vi "ProdaNG.Configurator.Popup.Delete.vi"(10 "Elements to delete":T1[](array[typedef])) -> (5 "OK?":bool)   [LabVIEW 2016]
uses:
  ProdaNG.Tree.Fglb.Data.ctl
  ProdaNG.Tree.Fglb.Element.ctl
panel:
  out "unblock time":timestamp
  in  "Button.Cancel":bool
  in  "Button.OK":bool
  out "Msg":string
  out "Elements":i32(listbox)
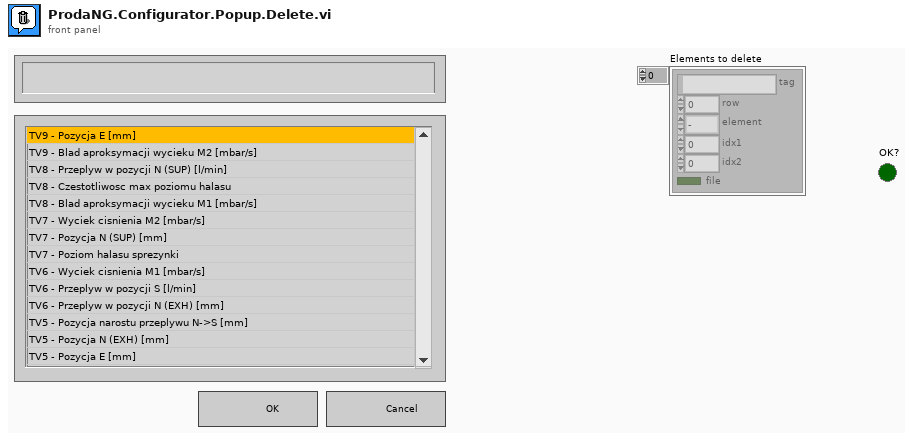
[diagram p1: front panel]
types:
  T1 = typedef "ProdaNG.Tree.Fglb.Data.ctl" = cluster{"tag":string, "row":i32, "element":T2, "idx1":i32, "idx2":i32, "file":bool}
  T2 = typedef "ProdaNG.Tree.Fglb.Element.ctl" = enum16{"-", "PP", "TS", "TP", "TV"}
  T3 = enum8{"Enabled", "Disabled", "Disabled and Grayed Out"}
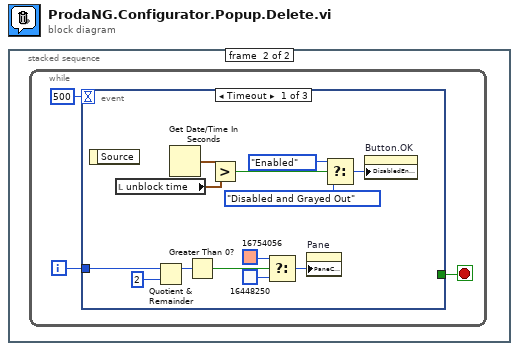
[diagram p0: block diagram]
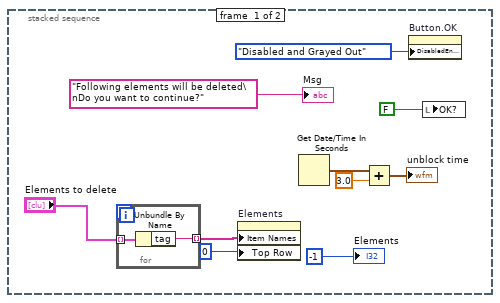
[diagram p2: hidden frame]
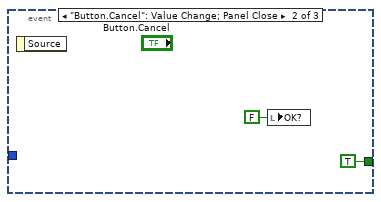
[diagram p3: hidden frame]
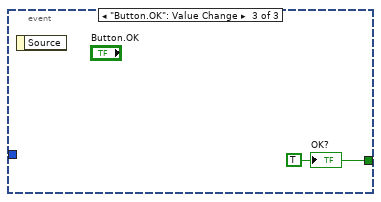
[diagram p4: hidden frame]
diagram:
  n1 = stacked-sequence {
    frame #0 {
      n2 = for {
        tunnel: "Elements to delete" -> [w12] mode=indexing
        tunnel: [w11] -> w7 mode=indexing
        n3 = Unbundle By Name(w12) -> ("tag"=w11:string)
      }
      n4 = property on="Elements" class="LstBox (strict)"("Item Names"=w7, "Top Row"=0) -> ()  [unwired: 2 in, 2 out]
      n5 = Get Date/Time In Seconds() -> (seconds since 1Jan1904=w3:timestamp)
      n6 = Add(x=w3, y=3.0) -> (x+y=→"unblock time":timestamp)
      n7 = property on="Button.OK" class="Bool"("DisabledEnum"=T3."Disabled and Grayed Out" ("Disabled")) -> ()  [unwired: 2 in, 2 out]
      n8 = local write "OK?"(FALSE ("OK?")) -> ()
      "Msg" <- "Following elements will be deleted\nDo you want to continue?" ("Msg")
      "Elements" <- -1 ("Elements")
    }
    frame #1 {
      n9 = while {
        i -> [w13]
        stop <- w15 stop-if-true
        n10 = event shown="[0] Timeout" {
          selector: _ -> [_ _ _]
          dyn-events: _ -> [_ _ _]
          timeout: 500 -> [_ _ _]
          tunnel: [_ TRUE ("OK?") w31] -> w15
          tunnel: w13 -> [w28 _ _]
          event Timeout {
            n11 = event-data() -> ()  [unwired: 1 in, 1 out]
            n12 = local read "unblock time"() -> (w21:timestamp)
            n13 = Quotient & Remainder(x=w28, y=2) -> (x-y*floor(x/y)=w26:i32)  [unwired: 1 out]
            n14 = Get Date/Time In Seconds() -> (seconds since 1Jan1904=w20:timestamp)
            n15 = Greater Than 0?(x=w26) -> (x > 0?=w25:bool)
            n16 = Greater?(x=w20, y=w21) -> (0:w19:bool)
            n17 = Select(t=u32 16754056, s=w25, f=u32 16448250) -> (s? t:f=w22:u32)
            n18 = property on="Pane" class="Pane"("PaneColor"=w22) -> ()  [unwired: 2 in, 2 out]
            n19 = Select(t=T3."Enabled" ("Disabled"), s=w19, f=T3."Disabled and Grayed Out" ("Disabled")) -> (s? t:f=w18:T3)
            n20 = property on="Button.OK" class="Bool"("DisabledEnum"=w18) -> ()  [unwired: 2 in, 2 out]
          }
          event "Button.Cancel": Value Change; Panel Close {
            n21 = event-data() -> ()  [unwired: 1 in, 1 out]
            n22 = local write "OK?"(FALSE ("OK?")) -> ()
          }
          event "Button.OK": Value Change {
            w31 = TRUE ("OK?")
            n23 = event-data() -> ()  [unwired: 1 in, 1 out]
            "OK?" <- w31
          }
        }
      }
    }
  }
